vi "Periodic Tasks Test.vi"(8 "error in":errorcluster) -> ()   [LabVIEW 2015]
doc: "This VI runs in parallel to other tasks. It can contain as many user-defined periodic loops as you need. These can carry out PID or other sorts of timed response."
uses:
  Robot Global Data.vi
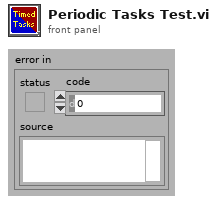
[diagram p1: front panel]
types:
  T1 = typedef "WPI_SerialPortRef.ctl" = cluster{"DevStatus":errorcluster, "Serial Port Name":refnum<visa-resource-name>}
  T2 = cluster{"Distance":dbl, "Angle":dbl, "x":dbl, "y":dbl}
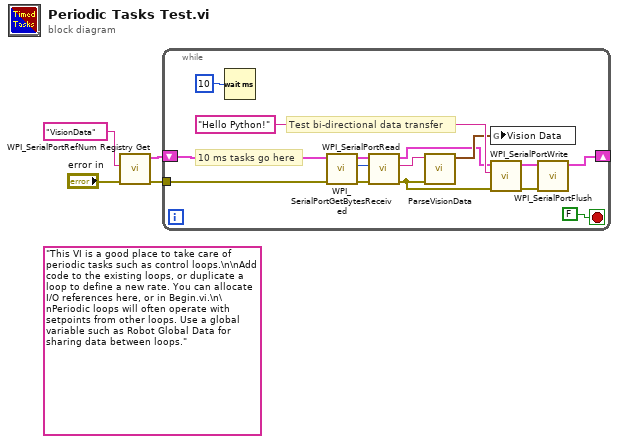
[diagram p0: block diagram]
diagram:
  (unwired) "This VI is a good place to take care of periodic tasks such as control loops.\n\nAdd code to the existing loops, or duplicate a loop to define a new rate. You can allocate I/O references here, or in Begin.vi.\n\nPeriodic loops will often operate with setpoints from other loops. Use a global variable such as Robot Global Data for sharing data between loops."
  n1 = call <vilib>:"WPI_SerialPortRefNum Registry Get.vi"("error in (no error)"="error in", "refnum name"="VisionData") -> ("error out"=w2:errorcluster, "SerialPortRef"=w1:T1)  [unwired: 8 in]
  n2 = while {
    tunnel: w2 -> [w7]
    shift-right: [w5] -> _
    shift-left: w1 -> [w6]
    stop <- FALSE stop-if-true
    # "Test bi-directional data transfer"
    # "10 ms tasks go here"
    n3 = Wait (ms)(milliseconds to wait=u32 10) -> ()  [unwired: 1 out]
    n4 = call <vilib>:"WPI_SerialPortGetBytesReceived.vi"("error in (no error)"=w7, "SerialPortRef"=w6) -> ("error out"=w15:errorcluster, "Bytes at Port"=w17:u32, "SerialPortRef"=w16:T1)  [unwired: 7 in]
    n5 = call <vilib>:"WPI_SerialPortRead.vi"("error in (no error)"=w15, "Num Bytes to Read"=w17, "SerialPortRef"=w16) -> ("error out"=w9:errorcluster, "Buffer"=w11:string, "SerialPortRef"=w8:T1)  [unwired: 6 in]
    n6 = call "ParseVisionData.vi"("error in (no error)"=w9, "JSON String"=w11) -> ("Distance and Angle"=w10:T2)  [unwired: 8 in, 1 out]
    n7 = global write "Robot Global Data.vi" "Vision Data"(w10) -> ()
    n8 = call <vilib>:"WPI_SerialPortWrite.vi"("error in (no error)"=w9, "Buffer"="Hello Python!", "SerialPortRef"=w8) -> ("error out"=w13:errorcluster, "SerialPortRef"=w12:T1)  [unwired: 6 in, 1 out]
    n9 = call <vilib>:"WPI_SerialPortFlush.vi"("error in (no error)"=w13, "SerialPortRef"=w12) -> ("SerialPortRef"=w5:T1)  [unwired: 8 in, 1 out]
  }
